vi "EIP Get Tag Info.vi"(8 "error in":errorcluster, 10 "Specified Channel Ref List":T1[](array[typedef]) format="%.0x", 11 "Item Ref in":T1 format="%.0x") -> (0 "error out":errorcluster, 2 "Tag Data":T2[](array[typedef]) {"Device Reference" format="%.0x"}, 3 "Item Ref out":T1 format="%.0x")   [LabVIEW 2011, in "Ethernet IP Custom Device Custom Device.lvlib"]
uses:
  Ethernet IP Custom Device Custom Device.lvlib
  <vilib>/NI Veristand/Custom Device API/Custom Device Item Ref.ctl
  EIP Tag Information.ctl
  <vilib>/NI Veristand/Custom Device API/Custom Device Item Info.ctl
  L5K Data Types.ctl
  Ethernet IP Global Strings.vi
  <vilib>/NI Veristand/Custom Device API/Get Item Property (U16).vi
  <vilib>/NI Veristand/Custom Device API/Get Item Property (String).vi
  <vilib>/NI Veristand/Custom Device API/Custom Device API.lvlib
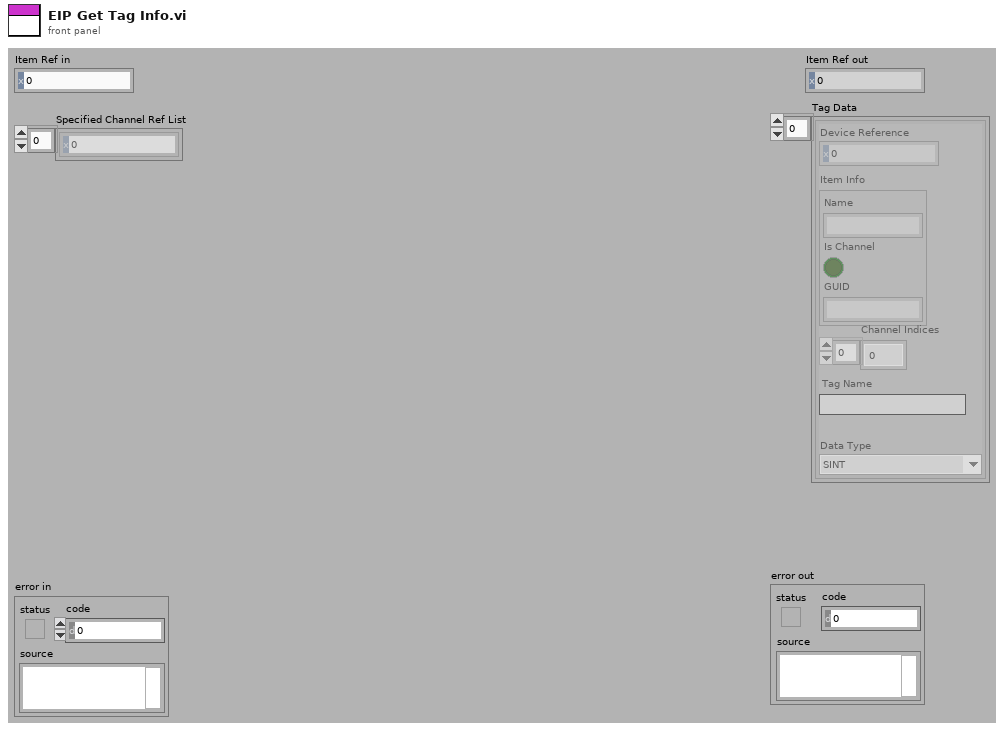
[diagram p1: front panel]
types:
  T1 = typedef "Custom Device API.lvlib/Custom Device Item Ref.ctl" = u64
  T2 = typedef "Ethernet IP Custom Device Custom Device.lvlib/EIP Tag Information.ctl" = cluster{"Item Info":T3, "Device Reference":T1, "Channel Indices":i32[], "Tag Name":string, "Data Type":T4}
  T3 = typedef "Custom Device API.lvlib/Custom Device Item Info.ctl" = cluster{"Name":string, "Is Channel":bool, "GUID":string}
  T4 = typedef "Ethernet IP Custom Device Custom Device.lvlib/L5K Data Types.ctl" = enum16{"SINT", "INT", "DINT", "REAL", "BOOL"}
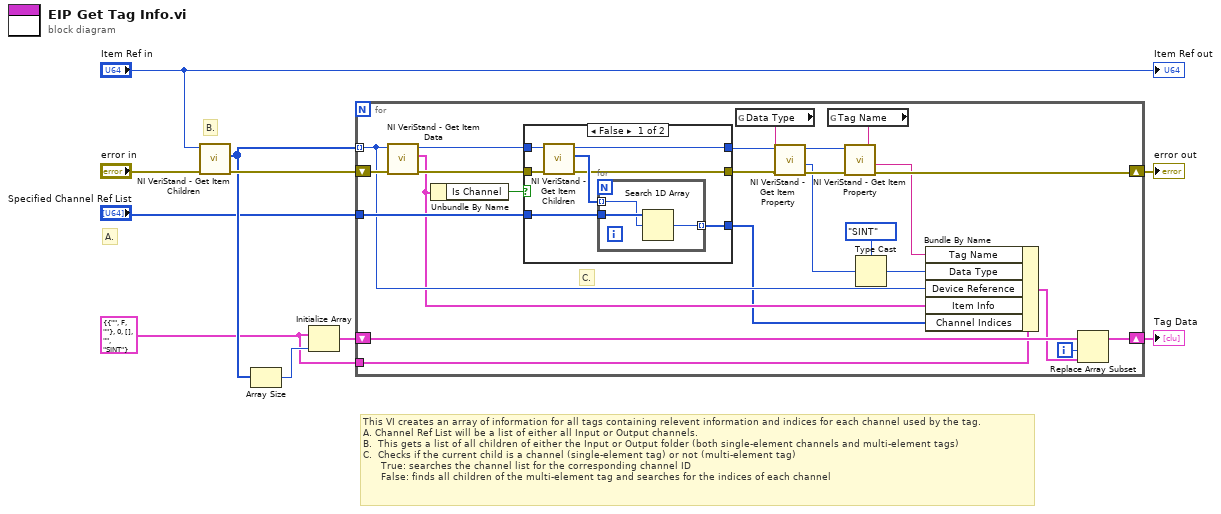
[diagram p0: block diagram]
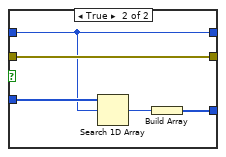
[diagram p2: hidden frame]
diagram:
  w3 = T2 {"Item Info"={"Name"="", "Is Channel"=FALSE, "GUID"=""}, "Device Reference"=0, "Channel Indices"=[], "Tag Name"="", "Data Type"=enum."SINT"} ("EIP Tag Information")
  # "B."
  # "A."
  # "This VI creates an array of information for all tags containing relevent information and indices for each channel used by the tag.\nA. Channel Ref List will be a list of either all Input or Output channels.\nB.  This gets a list of all children of either the Input or Output folder (both single-element channels and multi-element tags)\nC.  Checks if the current child is a channel (single-element tag) or not (multi-element tag)\n      True: searches the channel list for the corresponding channel ID \n      False: finds all children of the multi-element tag and searches for the indices of each channel"
  n1 = call <vilib>:"NI VeriStand - Get Item Children.vi"("error in (no error)"="error in", "Item Ref in"="Item Ref in") -> ("error out"=w10:errorcluster, "Child Refs"=w8:T1[])  [unwired: 6 in, 2 out]
  n2 = Array Size(array=w8) -> (size(s)=w7:i32)
  n3 = Initialize Array(w3, w7) -> (w6:T2[])
  n4 = for {
    tunnel: w8 -> [w26] mode=indexing
    tunnel: "Specified Channel Ref List" -> [w32]
    shift-right: [w17] -> w9
    shift-left: w10 -> [w31]
    shift-right: [w28] -> w2
    shift-left: w6 -> [w29]
    tunnel: w3 -> [w27]
    i -> [w22]
    # "C."
    n5 = call <vilib>:"NI VeriStand - Get Item Data.vi"("error in (no error)"=w31, "Item Ref in"=w26) -> ("error out"=w30:errorcluster, "Item Info"=w25:T3, "Item Ref out"=w33:T1)  [unwired: 6 in, 1 out]
    n6 = Unbundle By Name(w25) -> ("Is Channel"=w34:bool)
    n7 = case shown="False" w34 {
      tunnel: w33 -> [w41 w45]
      tunnel: w32 -> [w39 w49]
      tunnel: w30 -> [w38 w48]
      tunnel: [w36 w48] -> w20
      tunnel: [w37 w46] -> w24
      tunnel: [w35 w45] -> w19
      frame False {
        n8 = call <vilib>:"NI VeriStand - Get Item Children.vi"("error in (no error)"=w38, "Item Ref in"=w41) -> ("error out"=w36:errorcluster, "Child Refs"=w40:T1[], "Item Ref out"=w35:T1)  [unwired: 6 in, 1 out]
        n9 = for {
          tunnel: w40 -> [w43] mode=indexing
          tunnel: w39 -> [w44]
          tunnel: [w42] -> w37 mode=indexing
          n10 = Search 1D Array(1D array=w44, element=w43) -> (index of element=w42:i32)  [unwired: 1 in]
        }
      }
      frame True {
        n11 = Search 1D Array(1D array=w49, element=w45) -> (index of element=w47:i32)  [unwired: 1 in]
        n12 = Build Array(w47) -> (w46:i32[])
      }
    }
    n13 = global read "Ethernet IP Global Strings.vi" "Data Type"() -> (w12:string)
    n14 = call-poly <vilib>:"NI VeriStand - Get Item Property.vi"("error in (no error)"=w20, "Property Name"=w12, "Item Ref in"=w19) -> ("error out"=w21:errorcluster, "Value"=w14:u16, "Item Ref out"=w18:T1)  [unwired: 5 in, 1 out]
    n15 = global read "Ethernet IP Global Strings.vi" "Tag Name"() -> (w11:string)
    n16 = call-poly <vilib>:"NI VeriStand - Get Item Property.vi"("error in (no error)"=w21, "Property Name"=w11, "Item Ref in"=w18) -> ("error out"=w17:errorcluster, "Value"=w16:string)  [unwired: 5 in, 2 out]
    n17 = Type Cast(type=L5K_Data_Types."SINT" ("Data Type"), x=w14) -> (*(type *) &x=w15:T4)
    n18 = Bundle By Name(cluster=w27, "Tag Name"=w16, "Data Type"=w15, "Device Reference"=w26, "Item Info"=w25, "Channel Indices"=w24) -> (w23:T2)
    n19 = Replace Array Subset(array=w29, new element=w23, index=w22) -> (w28:T2[])
  }
  "error out" <- w9
  "Tag Data" <- w2
  "Item Ref out" <- "Item Ref in"
